vi "VerifyArguments.vi"(8 "error in (no error)":errorcluster, 11 "SaveForPrevious in":refnum<class "SaveForPrevious.lvclass">) -> (0 "error out":errorcluster, 3 "SaveForPrevious out":refnum<class "SaveForPrevious.lvclass">)   [LabVIEW 2014, in "SaveForPrevious.lvclass"]
doc: "Ensures required arguments are provided to the LabVIEWCLI."
uses:
  SaveForPrevious.lvclass
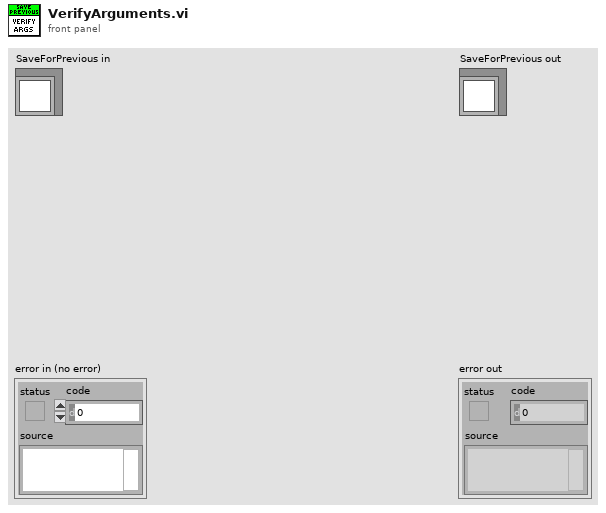
[diagram p1: front panel]
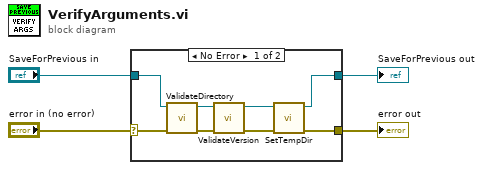
[diagram p0: block diagram]
diagram:
  n1 = case shown="No Error" "error in (no error)" {
    selector: "error in (no error)" -> [w12 w14]
    tunnel: [w7 w14] -> w3
    tunnel: [w5 w13] -> w1
    tunnel: "SaveForPrevious in" -> [w8 w13]
    frame No Error {
      n2 = call "ValidateDirectory.vi"("error in (no error)"=w12, "SaveForPrevious in"=w8) -> ("error out"=w11:errorcluster, "SaveForPrevious out"=w9:refnum<class "SaveForPrevious.lvclass">)  [unwired: 8 in]
      n3 = call "ValidateVersion.vi"("error in (no error)"=w11, "SaveForPrevious in"=w9) -> ("error out"=w10:errorcluster, "SaveForPrevious out"=w6:refnum<class "SaveForPrevious.lvclass">)  [unwired: 8 in]
      n4 = call "SetTempDir.vi"("error in (no error)"=w10, "SaveForPrevious in"=w6) -> ("error out"=w7:errorcluster, "SaveForPrevious out"=w5:refnum<class "SaveForPrevious.lvclass">)  [unwired: 8 in]
    }
    frame Error {
    }
  }
  "error out" <- w3
  "SaveForPrevious out" <- w1
